vi "Read server params.vi"(8 "error in (no error)":errorcluster, 11 "RESTLoaderBase in":refnum<class "RESTLoaderBase.lvclass">) -> (0 "error out":errorcluster, 2 "Server config":T1={"API Root"="", "verify server"=FALSE, "Version (no version)"="", "Port (protocol specific)"=0, "Base URL"="", "Auth type"=enum."Token", "Auth string"="", "timeout (10000)"=10000, "Token preamble (Token)"="", "Token header key (Authorization)"=""}, 3 "RESTLoaderBase out":refnum<class "RESTLoaderBase.lvclass">)   [LabVIEW 2019, in "ByteREST.lvlib" / "RESTLoaderBase.lvclass"]
uses:
  RESTLoaderBase.lvclass
  ServerParams.ctl
  ByteRESTClass/ByteRESTBase/Auth/Authentication_type.ctl
  RESTLoaderBase.lvclass/RESTLoaderBase.ctl
  ByteRESTClass/ByteRESTBase/RESTBase.lvclass
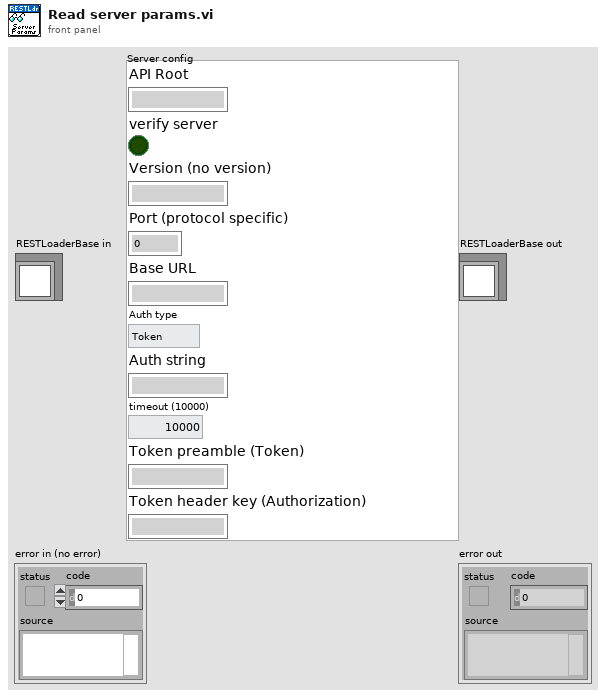
[diagram p1: front panel]
types:
  T1 = typedef "ByteREST.lvlib/RESTLoaderBase.lvclass/ServerParams.ctl" = cluster{"API Root":string, "verify server":bool, "Version (no version)":string, "Port (protocol specific)":u16, "Base URL":string, "Auth type":T2, "Auth string":string, "timeout (10000)":i32, "Token preamble (Token)":string, "Token header key (Authorization)":string}
  T2 = typedef "ByteREST.lvlib/RESTBase.lvclass/Authentication_type.ctl" = enum16{"Token"}
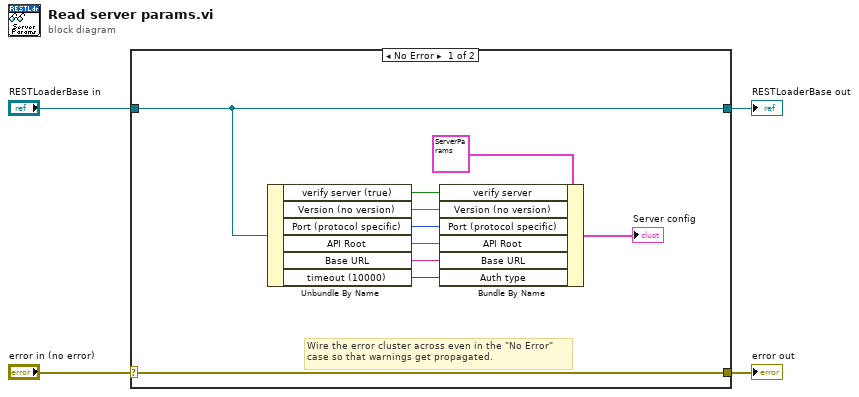
[diagram p0: block diagram]
diagram:
  n1 = case shown="No Error" "error in (no error)" {
    selector: "error in (no error)" -> [w14 w16]
    tunnel: [w14 w16] -> w3
    tunnel: [w13 w15] -> w1
    tunnel: "RESTLoaderBase in" -> [w13 w15]
    frame No Error {
      # "Wire the error cluster across even in the \"No Error\"\ncase so that warnings get propagated."
      n2 = Unbundle By Name(w13) -> ("verify server (true)"=w12:bool, "Version (no version)"=w11:string, "Port (protocol specific)"=w10:u16, "API Root"=w9:string, "Base URL"=w8:string, "timeout (10000)"=w5:i32)
      n3 = Bundle By Name(cluster=T1 {"API Root"="", "verify server"=FALSE, "Version (no version)"="", "Port (protocol specific)"=0, "Base URL"="", "Auth type"=enum."Token", "Auth string"="", "timeout (10000)"=10000, "Token preamble (Token)"="", "Token header key (Authorization)"=""} ("Server config"), "verify server"=w12, "Version (no version)"=w11, "Port (protocol specific)"=w10, "API Root"=w9, "Base URL"=w8, "Auth type"=w5) -> (→"Server config":T1)
    }
    frame Error {
    }
  }
  "error out" <- w3
  "RESTLoaderBase out" <- w1
